vi "Stepper Publish DAQ.vi"(8 "error in":errorcluster, 10 "BIBA 2017 Config":T7, 11 "Axis Data in":T1) -> (0 "error out":errorcluster, 3 "Axis Data out":T1)   [LabVIEW 2016, in "SMD-7615.lvlib"]
doc: "This VI reads Data (Digital Inputs, Motion I/O, Encoder Position & Velocity, ... ) of the specific Motor Device and publishes Data via corresponding Shared Variables."
uses:
  SMD-7615.lvlib
  CTL/Stepper Drive Config.ctl
  CTL/SV General.ctl
  CTL/SV Inputs.ctl
  CTL/SV Outputs.ctl
  CTL/Axis Data.ctl
  CTL/Motion IO.ctl
  CTL/Digital Lines (Read).ctl
  CTL/Status.ctl
  CTL/Encoder.ctl
  CTL/Position.ctl
  <vilib>/GPower/Error/Library/Append/AppendSingle.vi
  <vilib>/Utility/error.llb/Error Cluster From Error Code.vi
  <vilib>/ErrorRing/Error Ring.xnode
  <vilib>/GPower/Error/GPError.lvlib
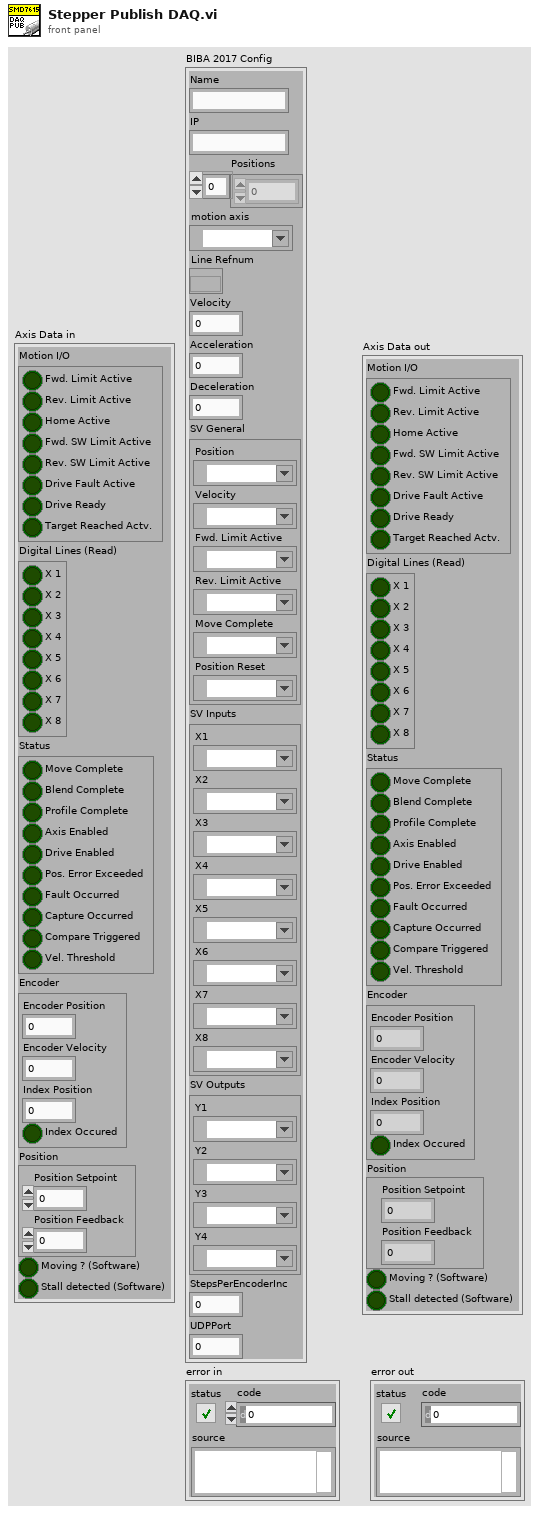
[diagram p1: front panel]
types:
  T1 = typedef "SMD-7615.lvlib/Axis Data.ctl" = cluster{"Motion I/O":T2, "Digital Lines (Read)":T3, "Status":T4, "Encoder":T5, "Position":T6, "Moving ? (Software)":bool, "Stall detected (Software)":bool}
  T2 = typedef "SMD-7615.lvlib/Motion IO.ctl" = cluster{"Fwd. Limit Active":bool, "Rev. Limit Active":bool, "Home Active":bool, "Fwd. SW Limit Active":bool, "Rev. SW Limit Active":bool, "Drive Fault Active":bool, "Drive Ready":bool, "Target Reached Actv.":bool}
  T3 = typedef "SMD-7615.lvlib/Digital Lines (Read).ctl" = cluster{"X 1":bool, "X 2":bool, "X 3":bool, "X 4":bool, "X 5":bool, "X 6":bool, "X 7":bool, "X 8":bool}
  T4 = typedef "SMD-7615.lvlib/Status.ctl" = cluster{"Move Complete":bool, "Blend Complete":bool, "Profile Complete":bool, "Axis Enabled":bool, "Drive Enabled":bool, "Pos. Error Exceeded":bool, "Fault Occurred":bool, "Capture Occurred":bool, "Compare Triggered":bool, "Vel. Threshold":bool}
  T5 = typedef "SMD-7615.lvlib/Encoder.ctl" = cluster{"Encoder Position":dbl, "Encoder Velocity":dbl, "Index Position":dbl, "Index Occured":bool}
  T6 = typedef "SMD-7615.lvlib/Position.ctl" = cluster{"Position Setpoint":dbl, "Position Feedback":dbl}
  T7 = typedef "SMD-7615.lvlib/Stepper Drive Config.ctl" = cluster{"Name":string, "IP":string, "Positions":dbl[], "motion axis ":refnum<k21>, "Line Refnum":refnum<k20>, "Velocity":dbl, "Acceleration":dbl, "Deceleration":dbl, "SV General":T8, "SV Inputs":T9, "SV Outputs":T10, "StepsPerEncoderInc":i32, "UDPPort":u16}
  T8 = typedef "SMD-7615.lvlib/SV General.ctl" = cluster{"Position":refnum<k21>, "Velocity":refnum<k21>, "Fwd. Limit Active":refnum<k21>, "Rev. Limit Active":refnum<k21>, "Move Complete":refnum<k21>, "Position Reset":refnum<k21>}
  T9 = typedef "SMD-7615.lvlib/SV Inputs.ctl" = cluster{"X1":refnum<k21>, "X2":refnum<k21>, "X3":refnum<k21>, "X4":refnum<k21>, "X5":refnum<k21>, "X6":refnum<k21>, "X7":refnum<k21>, "X8":refnum<k21>}
  T10 = typedef "SMD-7615.lvlib/SV Outputs.ctl" = cluster{"Y1":refnum<k21>, "Y2":refnum<k21>, "Y3":refnum<k21>, "Y4":refnum<k21>}
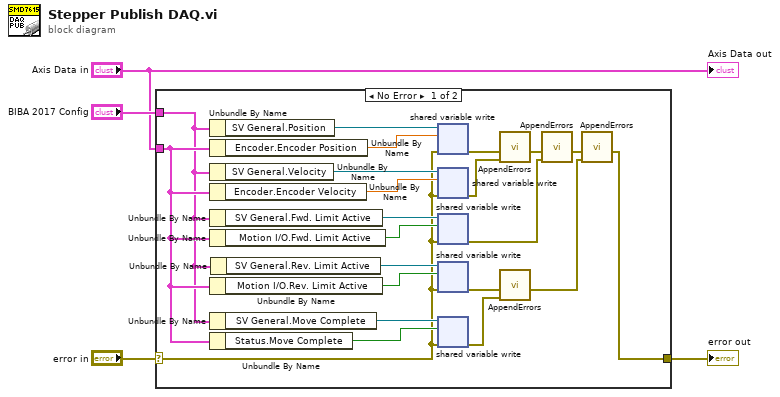
[diagram p0: block diagram]
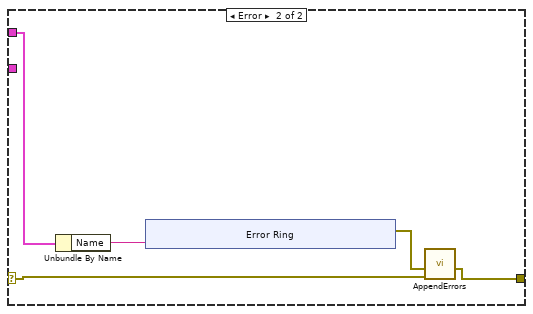
[diagram p2: hidden frame]
diagram:
  n1 = case shown="No Error" "error in" {
    selector: "error in" -> [w5 w28]
    tunnel: [w6 w27] -> w4
    tunnel: "BIBA 2017 Config" -> [w7 w31]
    tunnel: "Axis Data in" -> [w8 _]
    frame No Error {
      n2 = Unbundle By Name(w7) -> ("SV General.Position"=w9:refnum<k21>)
      n3 = Unbundle By Name(w8) -> ("Encoder.Encoder Position"=w10:dbl)
      n4 = Unbundle By Name(w7) -> ("SV General.Velocity"=w11:refnum<k21>)
      n5 = Unbundle By Name(w8) -> ("Encoder.Encoder Velocity"=w12:dbl)
      n6 = Unbundle By Name(w7) -> ("SV General.Fwd. Limit Active"=w13:refnum<k21>)
      n7 = Unbundle By Name(w8) -> ("Motion I/O.Fwd. Limit Active"=w14:bool)
      n8 = Unbundle By Name(w8) -> ("Motion I/O.Rev. Limit Active"=w16:bool)
      n9 = Unbundle By Name(w7) -> ("SV General.Move Complete"=w17:refnum<k21>)
      n10 = Unbundle By Name(w8) -> ("Status.Move Complete"=w18:bool)
      n11 = Unbundle By Name(w7) -> ("SV General.Rev. Limit Active"=w15:refnum<k21>)
      n12 = shared-variable-write(w9, w5, w10) -> (w20:errorcluster)  [unwired: 1 out]
      n13 = shared-variable-write(w11, w5, w12) -> (w21:errorcluster)  [unwired: 1 out]
      n14 = shared-variable-write(w13, w5, w14) -> (w22:errorcluster)  [unwired: 1 out]
      n15 = shared-variable-write(w15, w5, w16) -> (w23:errorcluster)  [unwired: 1 out]
      n16 = shared-variable-write(w17, w5, w18) -> (w24:errorcluster)  [unwired: 1 out]
      n17 = call-poly <vilib>:"AppendErrors.vi"("Error to append"=w21, "Error in"=w20) -> ("Appended errors out"=w19:errorcluster)  [unwired: 9 in]
      n18 = call-poly <vilib>:"AppendErrors.vi"("Error to append"=w24, "Error in"=w23) -> ("Appended errors out"=w26:errorcluster)  [unwired: 9 in]
      n19 = call-poly <vilib>:"AppendErrors.vi"("Error to append"=w22, "Error in"=w19) -> ("Appended errors out"=w25:errorcluster)  [unwired: 9 in]
      n20 = call-poly <vilib>:"AppendErrors.vi"("Error to append"=w26, "Error in"=w25) -> ("Appended errors out"=w6:errorcluster)  [unwired: 9 in]
    }
    frame Error {
      n21 = Unbundle By Name(w31) -> ("Name"=w30:string)
      n22 = xnode "Error Ring"("parameter 0"=w30) -> ("error out"=w29:errorcluster)
      n23 = call-poly <vilib>:"AppendErrors.vi"("Error to append"=w28, "Error in"=w29) -> ("Appended errors out"=w27:errorcluster)  [unwired: 9 in]
    }
  }
  "error out" <- w4
  "Axis Data out" <- "Axis Data in"
